vi "CDexperiment.vi"(2 "Error In":errorcluster, 4 "Зарядка-разрядка":T1, 5 "maximum output value":dbl=10.0 format="%0.2f") -> (0 "Error Out":errorcluster)   [LabVIEW 2012]
uses:
  <vilib>/DAQmx/create/channels.llb/DAQmx Create Channel (AI-Voltage-Basic).vi
  <vilib>/DAQmx/create/channels.llb/DAQmx Create Channel (AO-Voltage-Basic).vi
  <vilib>/DAQmx/configure/timing.llb/DAQmx Timing (Sample Clock).vi
  Charge Settings TypeDef.ctl
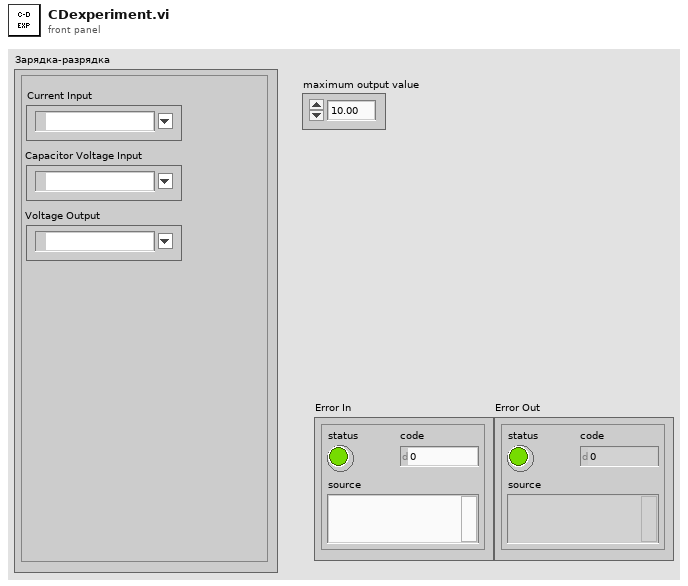
[diagram p1: front panel]
types:
  T1 = typedef "Charge Settings TypeDef.ctl" = cluster{"Current Input":tag, "Capacitor Voltage Input":tag, "Voltage Output":tag}
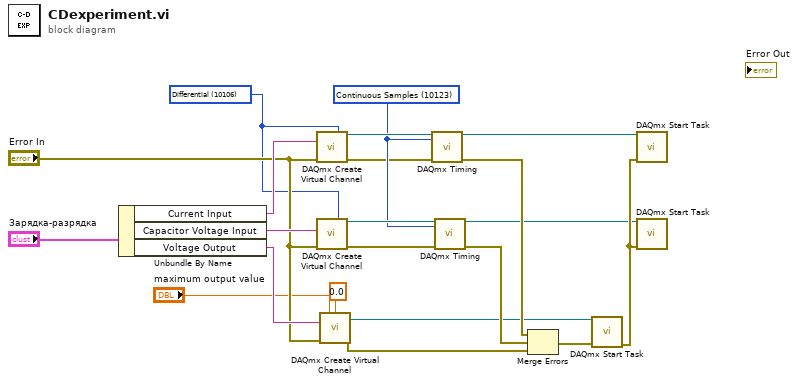
[diagram p0: block diagram]
diagram:
  w7 = 10106 items=["default"=-1, "RSE"=10083, "NRSE"=10078, "Differential"=10106, "Pseudodifferential"=12529] ("input terminal configuration")
  w15 = 10123 items=["Finite Samples"=10178, "Continuous Samples"=10123, "Hardware Timed Single Point"=12522] ("sample mode")
  n1 = Unbundle By Name("Зарядка-разрядка") -> ("Current Input"=w20:tag, "Capacitor Voltage Input"=w19:tag, "Voltage Output"=w18:tag)
  n2 = call-poly <vilib>:"DAQmx Create Virtual Channel.vi"("input terminal configuration"=w7, "physical channels"=w20, "error in"="Error In") -> ("task out"=w17:refnum<k21>, "error out"=w14:errorcluster)  [unwired: 11 in]
  n3 = call-poly <vilib>:"DAQmx Create Virtual Channel.vi"("input terminal configuration"=w7, "physical channels"=w19, "error in"="Error In") -> ("task out"=w16:refnum<k21>, "error out"=w13:errorcluster)  [unwired: 11 in]
  n4 = call-poly <vilib>:"DAQmx Create Virtual Channel.vi"("maximum value"="maximum output value", "minimum value"=0.0, "physical channels"=w18, "error in"="Error In") -> ("task out"=w8:refnum<k21>, "error out"=w9:errorcluster)  [unwired: 10 in]
  n5 = call-poly <vilib>:"DAQmx Timing.vi"("task/channels in"=w17, "sample mode"=w15, "error in"=w14) -> ("task out"=w2:refnum<k21>, "error out"=w11:errorcluster)  [unwired: 11 in]
  n6 = call-poly <vilib>:"DAQmx Timing.vi"("task/channels in"=w16, "sample mode"=w15, "error in"=w13) -> ("task out"=w1:refnum<k21>, "error out"=w10:errorcluster)  [unwired: 11 in]
  n7 = Merge Errors(w11, w10, w9) -> (w6:errorcluster)
  n8 = call <vilib>:"DAQmx Start Task.vi"("task/channels in"=w8, "error in"=w6) -> ("error out"=w3:errorcluster)  [unwired: 12 in, 1 out]
  n9 = call <vilib>:"DAQmx Start Task.vi"("task/channels in"=w2, "error in"=w3) -> ()  [unwired: 12 in, 2 out]
  n10 = call <vilib>:"DAQmx Start Task.vi"("task/channels in"=w1, "error in"=w3) -> ()  [unwired: 12 in, 2 out]
